vi "Adams Connect.vi"(0 "Module Address":string="localhost", 5 "Port":u16=502, 7 "connect timeout ms":i32=10000, 11 "error in (no error)":errorcluster) -> (4 "Module Ref":refnum<class "Modbus Master.lvclass">, 15 "error out":errorcluster)   [LabVIEW 2024]
doc: "Make a modbus master connection to Adams module slave."
uses:
  <vilib>/NI/Modbus Library/API/Master/Modbus Master.lvclass
  <vilib>/NI/Modbus Library/API/Wrapper/Create TCP Master.vi
  <vilib>/NI/Modbus Library/API/Wrapper/API Main.lvlib
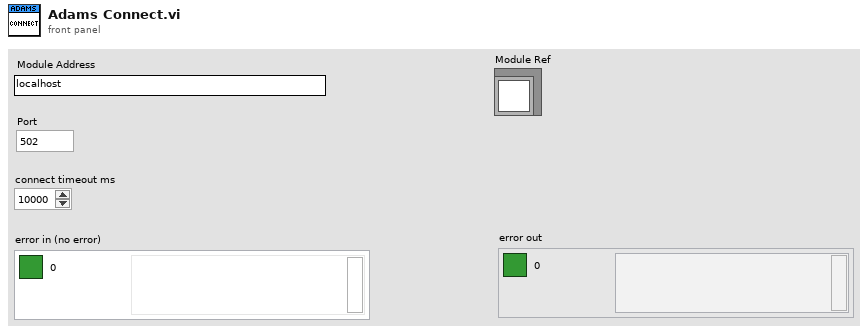
[diagram p1: front panel]
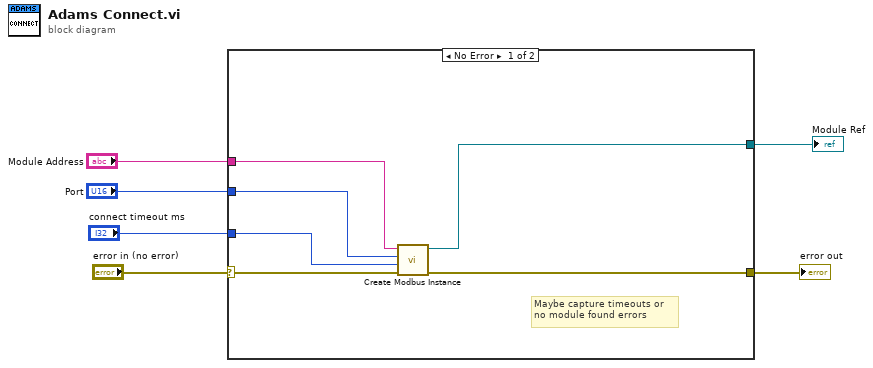
[diagram p0: block diagram]
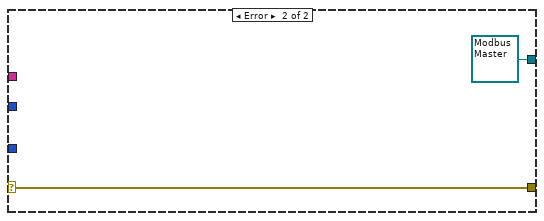
[diagram p2: hidden frame]
diagram:
  n1 = case shown="No Error" "error in (no error)" {
    selector: "error in (no error)" -> [w10 w14]
    tunnel: "Module Address" -> [w12 _]
    tunnel: "Port" -> [w11 _]
    tunnel: "connect timeout ms" -> [w9 _]
    tunnel: [w8 w14] -> w2
    tunnel: [w7 refnum<class "Modbus Master.lvclass"> refnum ("TCP master instance")] -> w1
    frame No Error {
      # "Maybe capture timeouts or\nno module found errors"
      n2 = call-poly <vilib>:"Create Modbus Instance.vi"("error in"=w10, "connect timeout ms"=w9, "port (502)"=w11, "address"=w12) -> ("error out"=w8:errorcluster, "TCP master instance"=w7:refnum<class "Modbus Master.lvclass">)  [unwired: 6 in]
    }
    frame Error {
    }
  }
  "error out" <- w2
  "Module Ref" <- w1
